vi "alignment3.vi"() -> ()   [LabVIEW 2020]
uses:
  <vilib>/DAQmx/read.llb/DAQmx Read (Counter 1D U32 1Chan NSamp).vi
  <vilib>/DAQmx/create/channels.llb/DAQmx Create Channel (CI-Period).vi
  <vilib>/DAQmx/configure/timing.llb/DAQmx Timing (Implicit).vi
  <vilib>/DAQmx/create/channels.llb/DAQmx Create Channel (CO-Pulse Generation-Frequency).vi
  <vilib>/DAQmx/miscellaneous.llb/DAQmx Fill In Error Info.vi
  <resource>/objmgr/daqmx.rc
  <vilib>/Analysis/NI_AALBase.lvlib
panel:
  out "deleted portion":u32[](array[numeric])
  out "array w/ subset deleted":u32[](array[numeric])
  out "Loop Time (ms) 2":u32=10
  out "sd":u32=4999
  out "mean":dbl(graph)
  out "data":u32[](graph)
  out "Input.BufSize":u32=1000000 format="%.0p"
  out "InSize 2":i32=5000 caption="Received Array size"
  out "max value 2":u32=1251317704
  out "min value 2":u32=4999
  out "Consumer Iteration 2":i32=1109257
  in  "stop 3":bool
  in  "number of samples per channel 2":i32=5000
  out "Producer Iteration 2":i32=1109256
  out "error out 2":errorcluster
  in  "dwell time (ms)":dbl=1.0 format="%.6f"
  in  "Photon Input (PFI)":tag="/Dev1/PFI0"
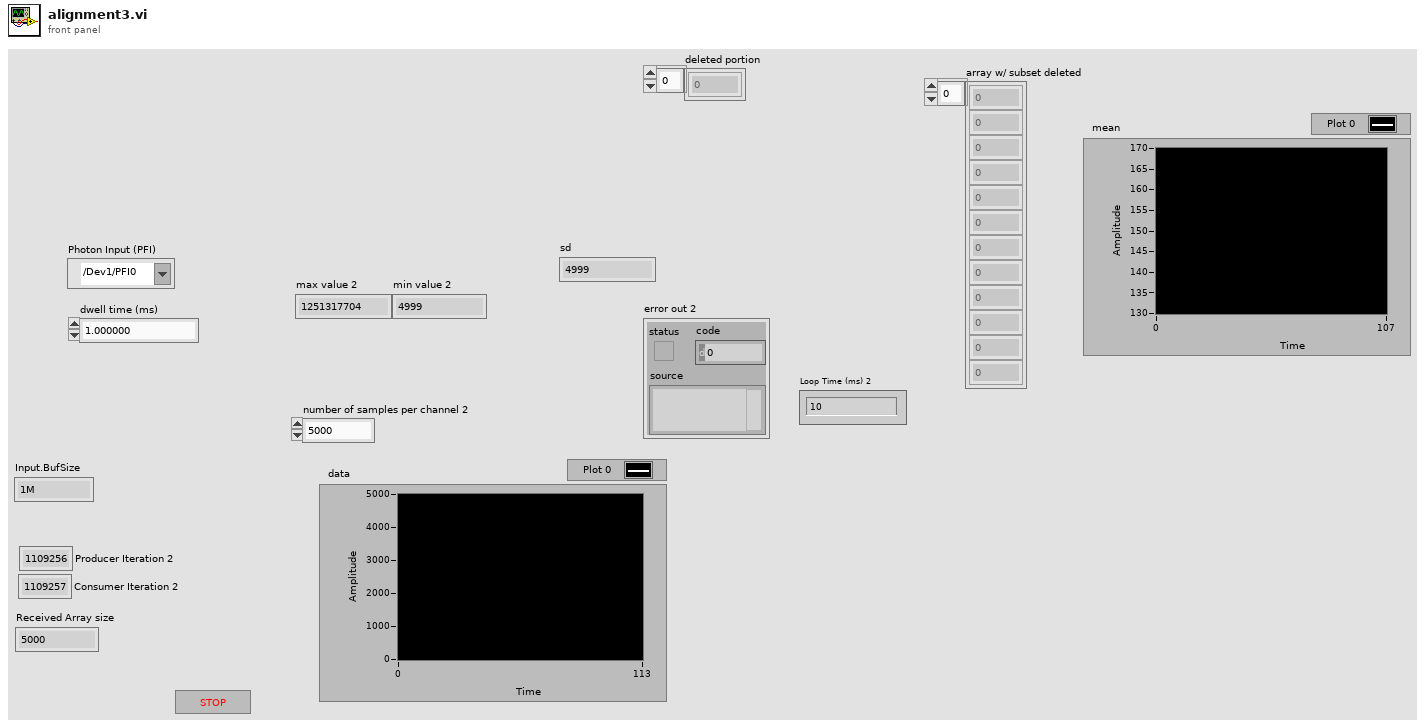
[diagram p1: front panel]
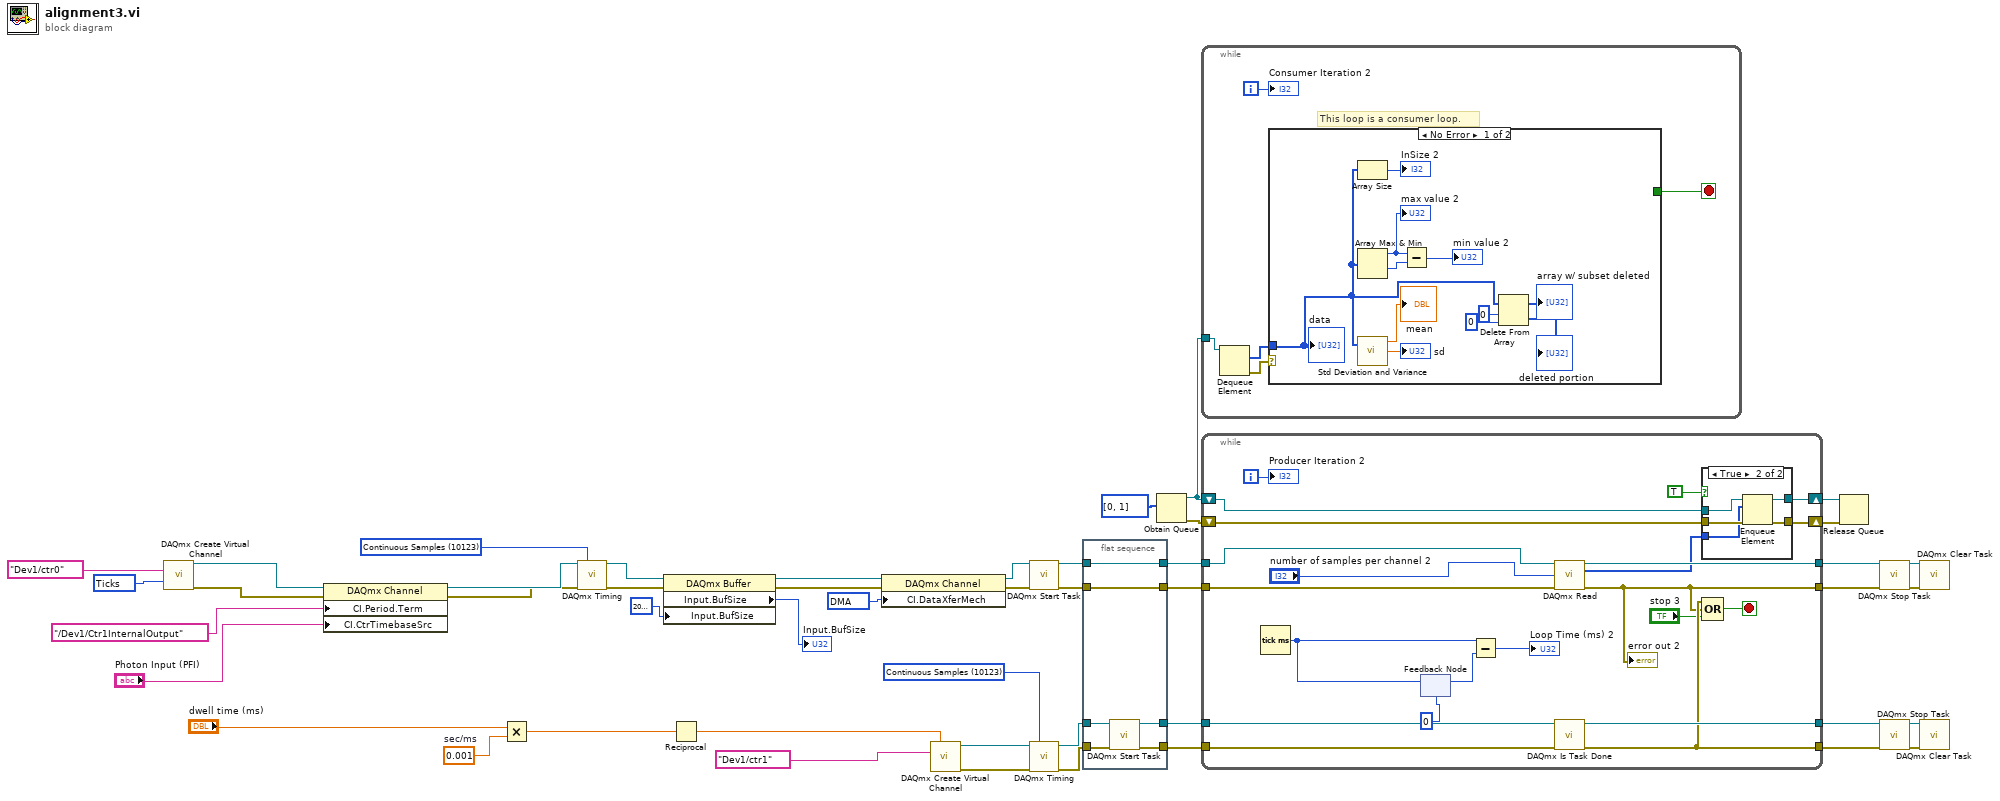
[diagram p0: block diagram]
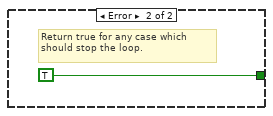
[diagram p2: hidden frame]
diagram:
  w9 = 10054 items=["DMA"=10054, "Interrupts"=10204, "Programmed I/O"=10264, "USB Bulk"=12590] ("CI.DataXferMech")
  w29 = 0.001  # sec/ms
  w39 = 10304 items=["Seconds"=10364, "Ticks"=10304, "From Custom Scale"=10065] ("units")
  w40 = 10123 items=["Finite Samples"=10178, "Continuous Samples"=10123, "Hardware Timed Single Point"=12522] ("sample mode")
  w41 = 10123 items=["Finite Samples"=10178, "Continuous Samples"=10123, "Hardware Timed Single Point"=12522] ("sample mode")
  n1 = call-poly <vilib>:"DAQmx Create Virtual Channel.vi"("counter"=tag "Dev1/ctr0", "units"=w39) -> ("task out"=w36:refnum<k21>, "error out"=w35:errorcluster)  [unwired: 12 in]
  n2 = property class="DAQmx Channel"(reference=w36, error in=w35, "CI.Period.Term"=tag "/Dev1/Ctr1InternalOutput", "CI.CtrTimebaseSrc"="Photon Input (PFI)") -> (reference out=w34:refnum<k21>, error out=w33:errorcluster)
  n3 = Multiply(x="dwell time (ms)", y=w29) -> (x*y=w28:dbl)
  n4 = call-poly <vilib>:"DAQmx Timing.vi"("task/channels in"=w34, "sample mode"=w40, "error in"=w33) -> ("task out"=w4:refnum<k21>, "error out"=w3:errorcluster)  [unwired: 11 in]
  n5 = property class="DAQmx Buffer"(reference=w4, error in=w3, "Input.BufSize"=u32 2000000 ("samples per channel")) -> (reference out=w8:refnum<k21>, error out=w6:errorcluster, "Input.BufSize"=→"Input.BufSize":u32)
  n6 = Reciprocal(x=w28) -> (1/x=w27:dbl)
  n7 = property class="DAQmx Channel"(reference=w8, error in=w6, "CI.DataXferMech"=w9) -> (reference out=w2:refnum<k21>, error out=w1:errorcluster)
  n8 = call-poly <vilib>:"DAQmx Create Virtual Channel.vi"("frequency"=w27, "counter"=tag "Dev1/ctr1") -> ("task out"=w46:refnum<k21>, "error out"=w47:errorcluster)  [unwired: 12 in]
  n9 = call <vilib>:"DAQmx Start Task.vi"("task/channels in"=w2, "error in"=w1) -> ("task out"=w26:refnum<k21>, "error out"=w25:errorcluster)  [unwired: 12 in]
  n10 = call-poly <vilib>:"DAQmx Timing.vi"("task/channels in"=w46, "sample mode"=w41, "error in"=w47) -> ("task out"=w45:refnum<k21>, "error out"=w44:errorcluster)  [unwired: 11 in]
  n11 = flat-sequence {
    tunnel: w45 -> [w53]
    tunnel: w44 -> [w52]
    tunnel: [w51] -> w12
    tunnel: [w50] -> w13
    tunnel: w26 -> [w48]
    tunnel: w25 -> [w49]
    tunnel: [w49] -> w15
    tunnel: [w48] -> w14
    frame #0 {
      n12 = call <vilib>:"DAQmx Start Task.vi"("task/channels in"=w53, "error in"=w52) -> ("task out"=w50:refnum<k21>, "error out"=w51:errorcluster)  [unwired: 12 in]
    }
  }
  n13 = Obtain Queue(element data type=u32[] [0, 1] ("data")) -> (queue out=w24:refnum<queue>, error out=w23:errorcluster)  [unwired: 4 in, 1 out]
  n14 = while {
    tunnel: w24 -> [w58]
    i -> [w54]
    stop <- w55 stop-if-true
    # "This loop is a consumer loop."
    n15 = Dequeue Element(queue=w58) -> (element=w56:u32[], error out=w57:errorcluster)  [unwired: 2 in, 2 out]
    n16 = case shown="No Error" w57 {
      tunnel: w56 -> [w63 _]
      tunnel: [_ TRUE] -> w55
      frame No Error {
        n17 = Array Size(array=w63) -> (size(s)=→"InSize 2":i32)
        n18 = Array Max & Min(array=w63) -> (max value=w68:u32, min value=w67:u32)  [unwired: 2 out]
        "max value 2" <- w68
        n19 = call <vilib>:"Std Deviation and Variance.vi"("X"=w63) -> ("mean"=→"mean":dbl, "standard deviation"=→"sd":dbl)  [unwired: 1 in, 1 out]
        n20 = Subtract(x=w68, y=w67) -> (x-y=→"min value 2":u32)
        n21 = Delete From Array(array=w63, length=0, index=0) -> (deleted portion=→"deleted portion":u32[], array with subset deleted=→"array w/ subset deleted":u32[])
        "data" <- w63
      }
      frame Error {
        # "Return true for any case which should stop the loop."
      }
    }
    "Consumer Iteration 2" <- w54
  }
  n22 = while {
    shift-right: [w82] -> w21
    shift-left: w23 -> [w90]
    shift-right: [w91] -> w22
    shift-left: w24 -> [w92]
    tunnel: [w88] -> w18
    tunnel: [w77] -> w17
    tunnel: w15 -> [w87]
    tunnel: w14 -> [w86]
    tunnel: w13 -> [w81]
    tunnel: w12 -> [w80]
    tunnel: [w79] -> w11
    tunnel: [w78] -> w10
    i -> [w83]
    stop <- w75 stop-if-true
    n23 = Tick Count (ms)() -> (millisecond timer value=w74:u32)
    n24 = feedback #1(u32 0 ("millisecond timer value")) -> (w73:u32)
    n25 = feedback-in #1(w74) -> ()
    n26 = Subtract(x=w74, y=w73) -> (x-y=→"Loop Time (ms) 2":u32)
    n27 = call-poly <vilib>:"DAQmx Read.vi"("task/channels in"=w86, "number of samples per channel"="number of samples per channel 2", "error in"=w87) -> ("task out"=w88:refnum<k21>, "data"=w85:u32[], "error out"=w77:errorcluster)  [unwired: 10 in]
    "error out 2" <- w77
    n28 = call <vilib>:"DAQmx Is Task Done.vi"("task/channels in"=w81, "error in"=w80) -> ("task out"=w79:refnum<k21>, "error out"=w78:errorcluster)  [unwired: 11 in, 1 out]
    n29 = case shown="True" TRUE ("Case Constant\n(See Context Help)") {
      tunnel: w92 -> [w94 w99]
      tunnel: [w94 w98] -> w91
      tunnel: w90 -> [w93 w97]
      tunnel: [w93 w96] -> w82
      tunnel: w85 -> [_ w95]
      frame False {
      }
      frame True {
        n30 = Enqueue Element(queue=w99, element=w95, error in (no error)=w97) -> (queue out=w98:refnum<queue>, error out=w96:errorcluster)  [unwired: 1 in, 1 out]
      }
    }
    n31 = Compound Arithmetic op=OR(w78, w77, "stop 3") -> (w75:bool)
    "Producer Iteration 2" <- w83
  }
  n32 = Release Queue(queue=w22, error in (no error)=w21) -> ()  [unwired: 1 in, 3 out]
  n33 = call <vilib>:"DAQmx Stop Task.vi"("task/channels in"=w18, "error in"=w17) -> ("task out"=w19:refnum<k21>, "error out"=w20:errorcluster)  [unwired: 12 in]
  n34 = call <vilib>:"DAQmx Stop Task.vi"("task/channels in"=w11, "error in"=w10) -> ("task out"=w43:refnum<k21>, "error out"=w42:errorcluster)  [unwired: 12 in]
  n35 = call <vilib>:"DAQmx Clear Task.vi"("task in"=w19, "error in"=w20) -> ()  [unwired: 13 in, 1 out]
  n36 = call <vilib>:"DAQmx Clear Task.vi"("task in"=w43, "error in"=w42) -> ()  [unwired: 13 in, 1 out]
